vi "Skin_Tenting_Code_113018.vi"() -> ()   [LabVIEW 2017]
uses:
  <vilib>/Analysis/Matrix/Datatypes/RealMatrix.ctl
  <vilib>/Analysis/Matrix/NI_Matrix.lvlib
panel:
  out "Measurement Complete":bool
  out "Real Time Force Value":dbl
  in  "OK Button":bool caption="Start Test"
  in  "Measurement Location":string(combo) caption="Location of Measurement on Body"
  in  "Subject ID":string
  out "Force":dynamicdata(graph)
  out "Displacement":dynamicdata(graph)
  in  "Start Next Measurement":bool
  in  "Choose Save Folder Location":path
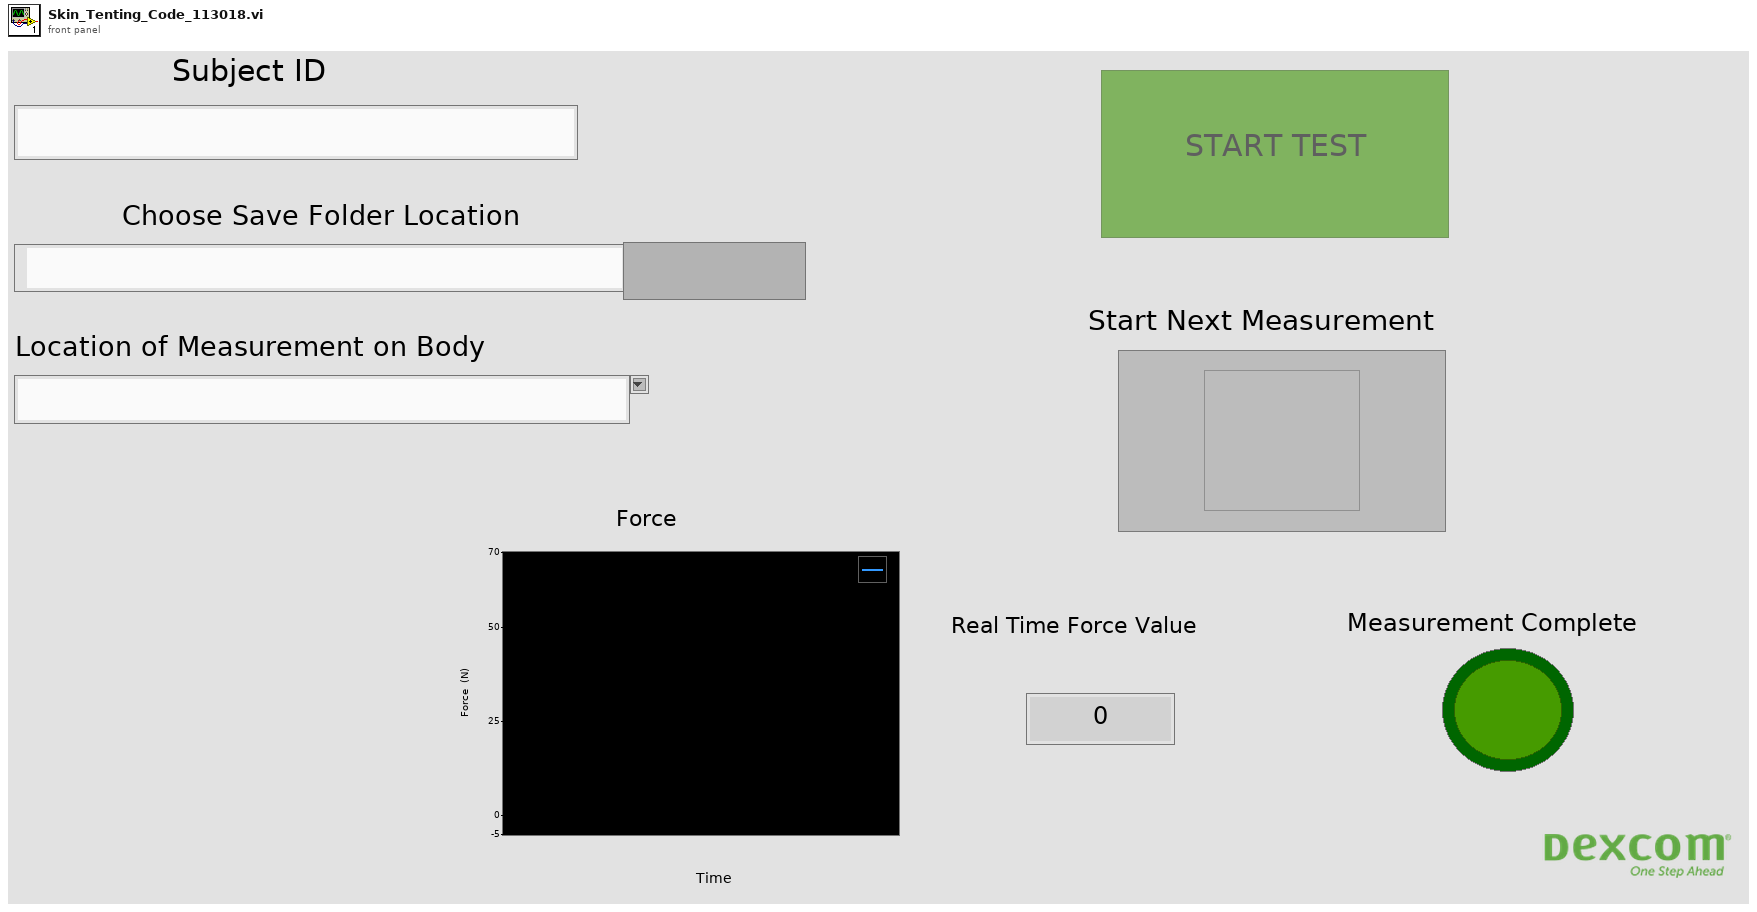
[diagram p1: front panel]
types:
  T1 = typedef "NI_Matrix.lvlib/RealMatrix.ctl" = dbl[][]
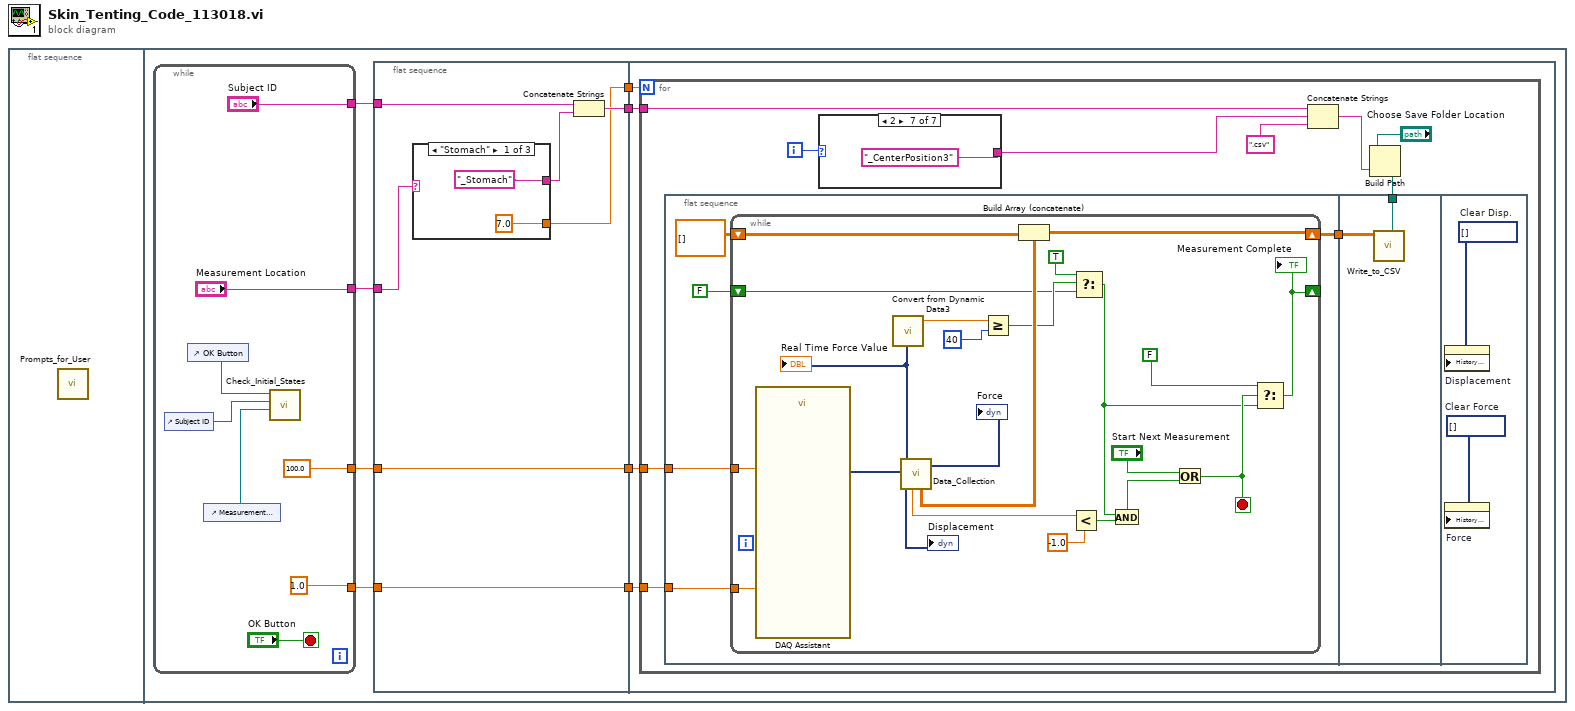
[diagram p0: block diagram]
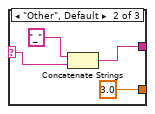
[diagram p2: hidden frame]
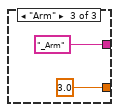
[diagram p3: hidden frame]
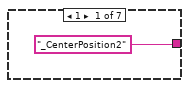
[diagram p4: hidden frame]
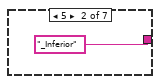
[diagram p5: hidden frame]
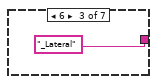
[diagram p6: hidden frame]
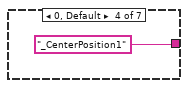
[diagram p7: hidden frame]
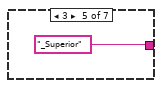
[diagram p8: hidden frame]
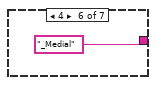
[diagram p9: hidden frame]
diagram:
  n1 = flat-sequence {
    frame #0 {
      n2 = call "Prompts_for_User.vi"() -> ()  [unwired: 12 in]
    }
    frame #1 {
      n3 = while {
        tunnel: ["Measurement Location"] -> w4
        tunnel: ["Subject ID"] -> w3
        tunnel: [1.0 ("Number of Samples per loop")] -> w2
        tunnel: [100.0 ("Rate of Acquisition")] -> w1
        stop <- "OK Button" stop-if-true
        n4 = control-ref of="Subject ID"() -> (w10:refnum<vi>)
        n5 = control-ref of="OK Button"() -> (w11:refnum<vi>)
        n6 = control-ref of="Measurement Location"() -> (w9:refnum<vi>)
        n7 = call "Check_Initial_States.vi"("CmbBox Refnum"=w9, "Str Refnum"=w10, "Boolean in"=w11) -> ()  [unwired: 9 in]
      }
      n8 = flat-sequence {
        tunnel: w3 -> [w21]
        tunnel: w2 -> [w22]
        tunnel: w1 -> [w23]
        tunnel: [w23] -> w8
        tunnel: [w22] -> w7
        tunnel: [w17] -> w6
        tunnel: [w20] -> w5
        tunnel: w4 -> [w19]
        tunnel: w8 -> [w35]
        tunnel: w7 -> [w34]
        tunnel: w6 -> [w33]
        tunnel: w5 -> [w32]
        frame #0 {
          n9 = case shown="\"Stomach\"" w19 {
            selector: w19 -> [_ w28 _]
            tunnel: [7.0 3.0 ("Numeric") 3.0] -> w17
            tunnel: ["_Stomach" w26 "_Arm"] -> w18
            frame "Stomach" {
            }
            frame "Other", Default {
              n10 = Concatenate Strings("_", w28) -> (w26:string)
            }
            frame "Arm" {
            }
          }
          n11 = Concatenate Strings(w21, w18) -> (w20:string)
        }
        frame #1 {
          n12 = for {
            N: w33 -> [_]
            tunnel: w35 -> [w44]
            tunnel: w34 -> [w43]
            tunnel: w32 -> [w42]
            i -> [w40]
            n13 = flat-sequence {
              tunnel: [w53] -> w45
              tunnel: w44 -> [w57]
              tunnel: w43 -> [w56]
              tunnel: w45 -> [w82]
              tunnel: w36 -> [w81]
              frame #0 {
                n14 = while {
                  shift-right: [w75] -> w53
                  shift-left: T1 [] ("Real Matrix") -> [w76]
                  tunnel: w57 -> [w79]
                  tunnel: w56 -> [w78]
                  shift-right: [w68] -> _
                  shift-left: FALSE ("t") -> [w70]
                  stop <- w65 stop-if-true
                  n15 = call "DAQ Assistant"("rate"=w79, "number of samples"=w78) -> ("data"=w80:dynamicdata)  [unwired: 14 in, 3 out]
                  n16 = call "Data_Collection.vi"("data"=w80) -> ("Scalar"=w63:dbl, "Force"=→"Force":dynamicdata, "Dynamic Data"=w74:dynamicdata, "Array"=w77:dbl[][], "Displacement"=→"Displacement":dynamicdata)  [unwired: 6 in]
                  "Real Time Force Value" <- w74
                  n17 = call "Convert from Dynamic Data3"("Dynamic Data Type"=w74) -> ("Scalar"=w73:dbl)  [unwired: 3 in]
                  n18 = Greater Or Equal?(x=w73, y=40) -> (x >= y?=w71:bool)
                  n19 = Build Array (concatenate)(w76, w77) -> (w75:T1)
                  n20 = Less?(x=w63, y=-1.0) -> (x < y?=w61:bool)
                  n21 = Select(t=TRUE, s=w71, f=w70) -> (s? t:f=w64:bool)
                  n22 = And(x=w64, y=w61) -> (x .and. y?=w60:bool)
                  n23 = Or(x="Start Next Measurement", y=w60) -> (x .or. y?=w65:bool)
                  n24 = Select(t=FALSE, s=w65, f=w64) -> (s? t:f=w68:bool)
                  "Measurement Complete" <- w68
                }
              }
              frame #1 {
                n25 = call "Write_to_CSV.vi"("appended path"=w81, "Real Matrix"=w82) -> ()  [unwired: 10 in]
              }
              frame #2 {
                w83 = dynamicdata[] []  # Clear Force
                w84 = dynamicdata[] []  # Clear Disp.
                n26 = property on="Displacement" class="WFChart (strict)"("History Data"=w84) -> ()  [unwired: 2 in, 2 out]
                n27 = property on="Force" class="WFChart (strict)"("History Data"=w83) -> ()  [unwired: 2 in, 2 out]
              }
            }
            n28 = case shown="2" w40 {
              tunnel: ["_CenterPosition2" "_Inferior" "_Lateral" "_CenterPosition1" "_Superior" "_Medial" "_CenterPosition3"] -> w39
              frame 1 {
              }
              frame 5 {
              }
              frame 6 {
              }
              frame 0, Default {
              }
              frame 3 {
              }
              frame 4 {
              }
              frame 2 {
              }
            }
            n29 = Concatenate Strings(w42, w39, ".csv") -> (w37:string)
            n30 = Build Path(base path="Choose Save Folder Location", name or relative path=w37) -> (appended path=w36:path)
          }
        }
      }
    }
  }
